vi "TorrosDown.vi"(9 "TorrosCurrPos":bool, 10 "TorrosButton":bool, 11 "ElevBasePosIn":T1) -> (2 "TorrosOut":bool, 3 "ElevBasePosOut":T1)   [LabVIEW 2018]
uses:
  ElevBasePos.ctl
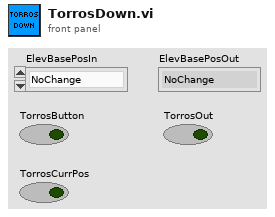
[diagram p1: front panel]
types:
  T1 = typedef "ElevBasePos.ctl" = enum16{"NoChange", "ShipHatch", "RocketHatch", "Carry", "Cargo"}
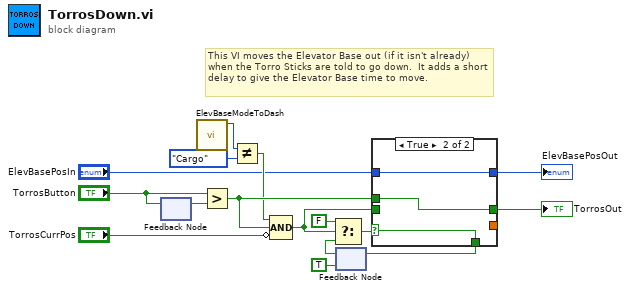
[diagram p0: block diagram]
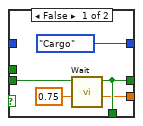
[diagram p2: hidden frame]
diagram:
  # "This VI moves the Elevator Base out (if it isn't already) when the Torro Sticks are told to go down.  It adds a short delay to give the Elevator Base time to move."
  n1 = feedback-in #1("TorrosButton") -> ()
  n2 = feedback #1() -> (w6:bool)  [unwired: 1 in]
  n3 = call "ElevBaseModeToDash.vi"() -> ("ElevBasePosOut"=w1:T1)  [unwired: 11 in]
  n4 = Greater?(x="TorrosButton", y=w6) -> (0:w8:bool)
  n5 = Not Equal?(x=w1, y=ElevBasePos."Cargo" ("f")) -> (x != y?=w4:bool)
  n6 = Compound Arithmetic op=AND(w4, w8, invert "TorrosCurrPos") -> (w15:bool)
  n7 = feedback #2(TRUE ("Completed")) -> (w12:bool)
  n8 = Select(t=FALSE, s=w15, f=w12) -> (s? t:f=w14:bool)
  n9 = case shown="True" w14 {
    selector: w14 -> [_ w22]
    tunnel: w8 -> [_ w23]
    tunnel: [w18 w23] -> w10
    tunnel: [w18 w22] -> w13
    tunnel: w15 -> [w19 _]
    tunnel: "ElevBasePosIn" -> [_ w24]
    tunnel: [ElevBasePos."Cargo" ("f") w24] -> w16
    tunnel: [w17 _] -> _
    frame False {
      n10 = call "Wait.vi"("Target Time (s)"=0.75, "Start Timer?"=w19) -> ("ElapsedTime"=w17:dbl, "Completed"=w18:bool)  [unwired: 8 in]
    }
    frame True {
    }
  }
  "ElevBasePosOut" <- w16
  "TorrosOut" <- w10
  n11 = feedback-in #2(w13) -> ()
